vi "libstop_listen.vi"(8 "error in (no error)":errorcluster, 10 "Function":string, 11 "input":i32) -> (0 "error out":errorcluster)   [LabVIEW 2015]
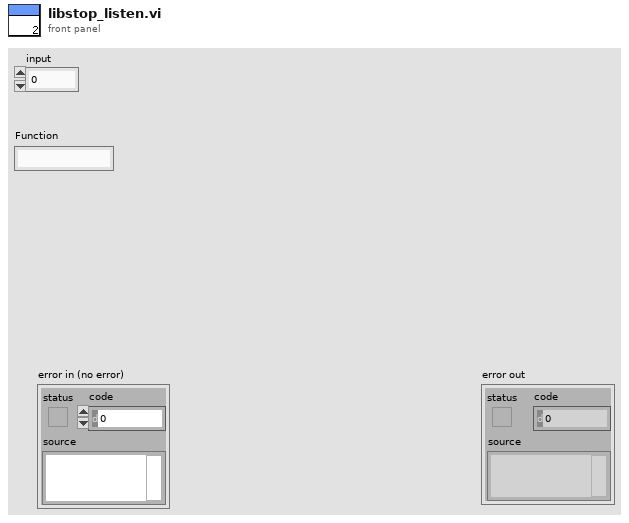
[diagram p1: front panel]
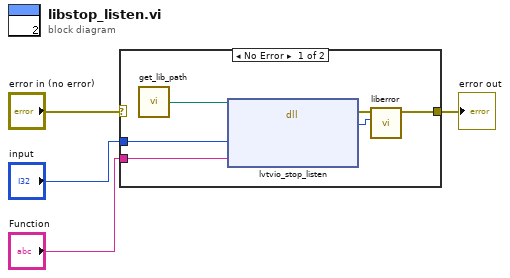
[diagram p0: block diagram]
diagram:
  n1 = case shown="No Error" "error in (no error)" {
    selector: "error in (no error)" -> [_ w11]
    tunnel: [w5 w11] -> w3
    tunnel: "Function" -> [w9 _]
    tunnel: "input" -> [w8 _]
    frame No Error {
      n2 = call "get_lib_path.vi"() -> ("Path"=w10:path)
      n3 = dll-call lib="S:/thingiverselv/lib/liblvtvio.dll" fn="lvtvio_stop_listen"(path in=w10, "input"=w8, "function"=w9) -> (error out=w7:errorcluster, "return type"=w6:i32)  [unwired: 4 in, 1 out]
      n4 = call "liberror.vi"("tvio errors"=w6, "error in (no error)"=w7) -> ("error out"=w5:errorcluster)  [unwired: 9 in]
    }
    frame Error {
    }
  }
  "error out" <- w3
